vi "Test_StartOfList_ReturnFirstItem.vi"(8 "error in (no error)":errorcluster, 11 "TestCase in":refnum<class "TestStringList.lvclass">) -> (0 "error out":errorcluster, 3 "TestCase out":refnum<class "TestStringList.lvclass">)   [LabVIEW 2015, in "StringList.lvlib" / "TestStringList.lvclass"]
uses:
  TestStringList.lvclass
  <vilib>/addons/_JKI Toolkits/VI Tester/TestCase.llb/TestCase.lvclass
  StringList.lvclass
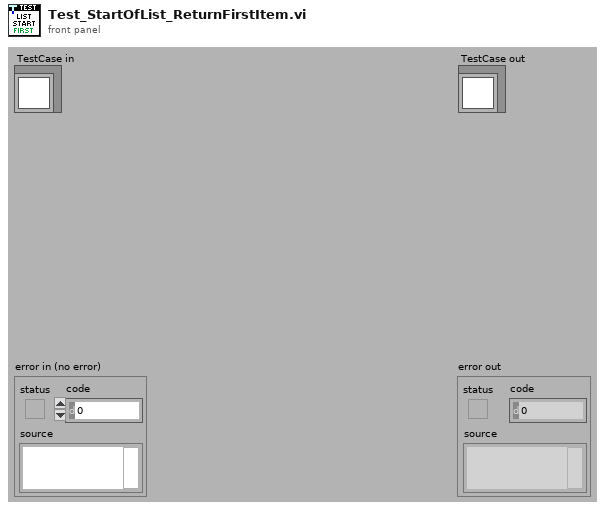
[diagram p1: front panel]
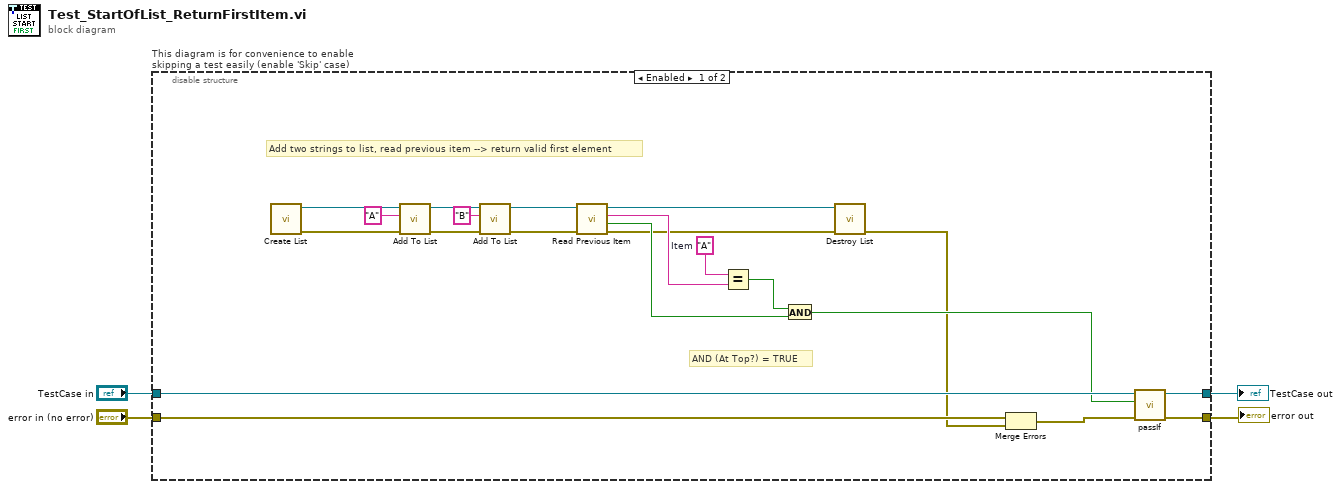
[diagram p0: block diagram]
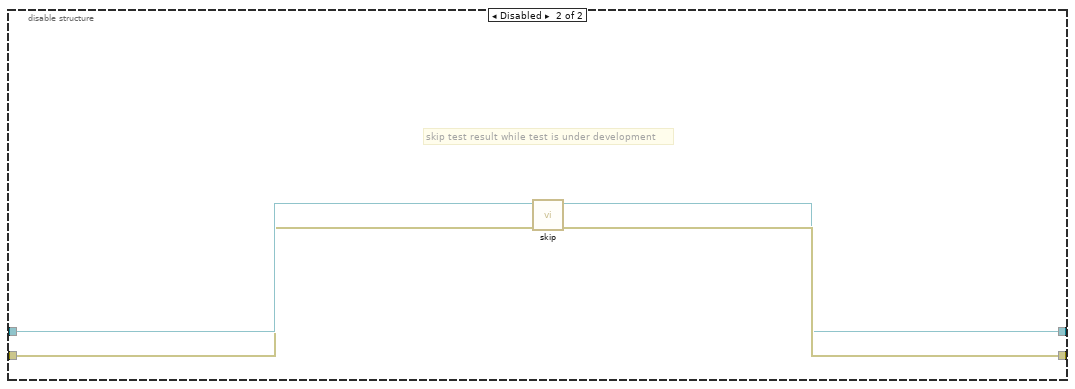
[diagram p2: hidden frame]
diagram:
  n1 = disable-structure "This diagram is for convenience to enable skipping a test easily (enable 'Skip' case)" shown="Enabled" {
    disable-tunnel: "TestCase in" -> [w25 w29]
    disable-tunnel: [w24 w27] -> w1
    disable-tunnel: [w23 w28] -> w3
    disable-tunnel: "error in (no error)" -> [w22 w26]
    frame Enabled {
      w16 = "A"  # Item
      # "AND (At Top?) = TRUE"
      # "Add two strings to list, read previous item --> return valid first element"
      n2 = call "Create List.vi"() -> ("error out"=w10:errorcluster, "StringList Reference"=w19:refnum<data-value>)  [unwired: 10 in]
      n3 = call "Add To List.vi"("error in (no error)"=w10, "Item"="A", "StringList Reference"=w19) -> ("error out"=w9:errorcluster, "StringList Reference"=w21:refnum<data-value>)  [unwired: 7 in]
      n4 = call "Add To List.vi"("error in (no error)"=w9, "Item"="B", "StringList Reference"=w21) -> ("error out"=w8:errorcluster, "StringList Reference"=w18:refnum<data-value>)  [unwired: 7 in]
      n5 = call "Read Previous Item.vi"("error in (no error)"=w8, "StringList Reference"=w18) -> ("error out"=w7:errorcluster, "At Top?"=w13:bool, "Item"=w15:string, "StringList Reference"=w11:refnum<data-value>)  [unwired: 6 in]
      n6 = Equal?(x=w16, y=w15) -> (x = y?=w14:bool)
      n7 = And(x=w14, y=w13) -> (x .and. y?=w12:bool)
      n8 = call "Destroy List.vi"("error in (no error)"=w7, "StringList Reference"=w11) -> ("error out"=w5:errorcluster)  [unwired: 8 in, 1 out]
      n9 = Merge Errors(w22, w5) -> (w6:errorcluster)
      n10 = call-dynamic "passIf.vi"("error in (no error)"=w6, "pass"=w12, "TestCase in"=w25) -> ("error out"=w23:errorcluster, "TestCase out"=w24:refnum<class "TestStringList.lvclass">)  [unwired: 7 in]
    }
    frame Disabled {
      # "skip test result while test is under development"
      n11 = call <vilib>:"skip.vi"("error in (no error)"=w26, "TestCase in"=w29) -> ("error out"=w28:errorcluster, "TestCase out"=w27:refnum<class "TestStringList.lvclass">)  [unwired: 8 in]
    }
  }
  "error out" <- w3
  "TestCase out" <- w1
